vi "Read Thermocouples and Voltages v181004_A.vi"() -> ()   [LabVIEW 2017]
doc: "I. Description:\nThis example demonstrates how to make continuous, hardware-timed temperature measurement using a thermocouple.\n\nII. Instructions for Running:\n1. Specify the Physical Channel where you have connected the thermocouple.\n2. Enter the Minimum and Maximum temperature values in degrees C you expect to measure. A smaller range will allow a more accurate measurement.\n3. Enter the scan rate at which you want to run the acquisition.\n4. Specify the type of thermocouple you are using.\n5. Thermocouple measurements require cold-junction compensation (CJC) to correctly scale them. Specify the source of your cold-junction compensation.\n6. If your CJC source is \"Internal\", skip the rest of the steps.\n7. If your CJC source is \"Constant Value\", specify the value (usually room temperature) in degrees C.\n8. If your CJC source is \"Channel\", specify the CJC Channel name. \n9. Specify the appropriate Auto Zero Mode. See your device's hardware manual to find out if your device supports this attribute.\n\nIII. Block Diagram Steps:\n1. Create a Thermocouple (TC) temperature measurement channel.\n2. Get all the channels in the task.\n3. Convert channel(s) array to a comma-delimited channel string.\n4. This attribute is set to compensate for input offset errors. May not be supported by all devices*.\n5. Call the Timing VI to specify the hardware timing parameters. Use device's internal clock, continuous mode acquisition and the sample rate specified by the user.\n6. Call the Start VI to program and start the acquisition.\n7. Read N samples and plot it. By default, the Read VI reads all available samples, but you can specify how many samples to read at a time and the timeout value. Continue reading data until the stop button is pressed or an error occurs. \n8. Call the Clear Task VI to clear the Task.\n9. Use the popup dialog box to display an error if any.\n\n* If your device does not support Auto Zero Mode bypass Step 2, 3, and 4.\n\nIV. I/O Connections Overview:\nConnect your thermocouple to the terminals corresponding to the Physical Channel I/O Control value."
uses:
  <vilib>/Utility/error.llb/DialogType.ctl
  <vilib>/DAQmx/read.llb/DAQmx Read (Counter 1D DBL 1Chan NSamp).vi
  <vilib>/Analysis/baseanly.llb/Mean (DBL).vi
  <vilib>/DAQmx/write.llb/DAQmx Write (Digital 1D Bool NChan 1Samp 1Line).vi
  <vilib>/DAQmx/read.llb/DAQmx Read (Analog 1D Wfm NChan NSamp).vi
  <vilib>/DAQmx/create/channels.llb/DAQmx Create Channel (AI-Voltage-Basic).vi
  <vilib>/DAQmx/configure/timing.llb/DAQmx Timing (Sample Clock).vi
  <vilib>/DAQmx/create/channels.llb/DAQmx Create Channel (DO-Digital Output).vi
  <vilib>/Waveform/WDTOps.llb/WDT Index Channel DBL.vi
  <vilib>/DAQmx/miscellaneous.llb/DAQmx Fill In Error Info.vi
  <vilib>/DAQmx/create/channels.llb/DAQmx Create Channel (CI-Period).vi
  <vilib>/DAQmx/configure/timing.llb/DAQmx Timing (Implicit).vi
  <vilib>/express/express arith-compare/Formula/XNode/ExpressFormulaBlockNode.xnode
  <resource>/objmgr/daqmx.rc
  <vilib>/Analysis/NI_AALBase.lvlib
  <vilib>/ptbypt/NI_PtbyPt.lvlib
panel:
  out "TRQ_T22_2SPD_INPUT_PULLEY":dbl=0.017996215820312494 format="%0.3f"
  in  "offset_TRQ_IN":dbl=-0.15 format="%5.2f"
  in  "(N·m)/V TRQ_IN":dbl=20.0 format="%5.2f"
  in  "CI.Period.DigFltr.MinPulseWidth":dbl=1e-05 format="%.3e"
  out "CALC_RPM_2SPD_IN_FV":dbl=3496.0559999999996 format="%0.1f"
  out "T2":dbl=102.18860626220703 format="%0.3f"
  in  "offset_T2":dbl=-50.0 format="%5.3f"
  in  "T2 °C/V":dbl=50.0 format="%5.3f"
  in  "offset RPM_IN":dbl=4.0 format="%5.2f"
  in  "RPM_OT/V":dbl=2803.738 format="%5.3f"
  out "RPM_2SPD_IN_FV":dbl=1.4714915466308593 format="%0.1f"
  in  "offset TRQ_OT":dbl format="%5.2f"
  in  "N·m/V":dbl=10.0 format="%5.2f"
  out "TRQ_2SPD_OT (N·m)":dbl=-0.0037994384765625 format="%0.3f"
  out "Power_OT (W)":dbl=-0.0009464121851047188 format="%.2f"
  in  "Physical Channel 2":tag="Dev2/ai0:7" caption="PCI-6143_2 Channels"
  out "rpm_out/rpm_in":dbl=1.6164955643487515 format="%.3g"
  out "switch_counts":dbl=4500000.0
  in  "switch_time (s)":dbl=900000.0
  out "AI Consumer Iterations":i32=21
  out "Counter Consumer":i32=248
  out "Counter Producer":i32=247
  out "PPR":i32=107
  out "Array":dbl[](array[numeric])
  out "Mean RPM_2SPD_OT":dbl
  out "data":dbl[][](array[numeric])
  in  "LV_CMD_2SPD_OIL_SLND":bool[](array[boolean])=[FALSE]
  in  "lines":tag="Dev1/port0/line0"
  out "RPM_2SPD_OT_6602":dbl format="%0.1f"
  in  "PPR Array":i32[](array[numeric])=[360, 107]
  in  "CI.Counter":tag[](array[tag])=["Dev3/ctr0", "Dev3/ctr1"]
  in  "CI.Period.Terminal":tag[](array[tag])=["/Dev3/PFI1", "/Dev3/PFI38"]
  in  "path":path=path "\\\\Achates.lan\\data/TeamShares/Testing Group/Bench Tests/PR22093 - Orthrus 2SpdSN3.4 Sprag Clutch durability testing/LabView Data"
  in  "DRVLN_PULLEY_RATIO":dbl=1.48 format="%.2f"
  out "delta-P":dbl=2.3032233810424803 format="%.3f"
  in  "F2 gpm/V":dbl=0.875 format="%5.3f"
  out "F2":dbl=0.5424336433410645 format="%0.3f"
  in  "offset_F2":dbl=-0.875 format="%5.3f"
  out "Recorded Blocks":dbl=-95911.0
  out "AI Producer Iterations":i32=20
  in  "Force Record":bool caption="Force Record Enable"
  out "RPM_DRVLN_6602":dbl format="%0.1f"
  in  "offset_RPM1":dbl format="%5.3f"
  in  "RPM_IN rpm/V":dbl=2362.2 format="%5.3f"
  out "RPM_2SPD_OT_FV":dbl=2.3786595581054684 format="%0.1f"
  in  "offset_T1":dbl=-50.0 format="%5.3f"
  in  "T1 °C/V":dbl=50.0 format="%5.3f"
  out "T1":dbl=104.08489227294922 format="%0.3f"
  out "P3":dbl=3.2324594879150386 format="%0.3f"
  in  "offset_P3":dbl=0.01 format="%5.3f"
  in  "P3 bar_g/V":dbl=2.05 format="%5.3f"
  out "P2":dbl=3.3167593002319333 format="%0.3f"
  in  "offset_P2":dbl format="%5.3f"
  in  "P2 bar_a/V":dbl=2.05 format="%5.3f"
  out "P1":dbl=1.013535919189453 format="%0.3f"
  in  "offset_P1":dbl=-0.01 format="%5.3f"
  in  "P1 bar_a/V":dbl=1.0 format="%5.3f"
  out "data 2":waveform(dbl)[](array[waveform])=[{"t0"=timestamp(3621514488.0231304 s since 1904-01-01), "dt"=0.1, "Y"=[-0.0004058837890625, 0.0021026611328125], "attributes"=variant("NI_ChannelName"=variant(string "Dev1/ai0"), "NI_UnitDescription"=variant(string "Volts"))}, {"t0"=timestamp(3621514488.0231304 s since 1904-01-01), "dt"=0.1, "Y"=[1.0246047973632812, 1.022467041015625], "attributes"=variant("NI_ChannelName"=variant(string "Dev1/ai0"), "NI_UnitDescription"=variant(string "Volts"))}, {"t0"=timestamp(3621514488.0231304 s since 1904-01-01), "dt"=0.1, "Y"=[1.6239944458007813, 1.6118682861328124], "attributes"=variant("NI_ChannelName"=variant(string "Dev1/ai0"), "NI_UnitDescription"=variant(string "Volts"))}, {"t0"=timestamp(3621514488.0231304 s since 1904-01-01), "dt"=0.1, "Y"=[1.5774093627929688, 1.5664535522460938], "attributes"=variant("NI_ChannelName"=variant(string "Dev1/ai0"), "NI_UnitDescription"=variant(string "Volts"))}, {"t0"=timestamp(3621514488.0231304 s since 1904-01-01), "dt"=0.1, "Y"=[3.0814483642578123, 3.0819473266601562], "attributes"=variant("NI_ChannelName"=variant(string "Dev1/ai0"), "NI_UnitDescription"=variant(string "Volts"))}, {"t0"=timestamp(3621514488.0231304 s since 1904-01-01), "dt"=0.1, "Y"=[1.62095947265625, 1.6188888549804688], "attributes"=variant("NI_ChannelName"=variant(string "Dev1/ai0"), "NI_UnitDescription"=variant(string "Volts"))}, {"t0"=timestamp(3621514488.0231304 s since 1904-01-01), "dt"=0.1, "Y"=[-0.018182373046875, -0.01845550537109375], "attributes"=variant("NI_ChannelName"=variant(string "Dev1/ai0"), "NI_UnitDescription"=variant(string "Volts"))}, {"t0"=timestamp(3621514488.0231304 s since 1904-01-01), "dt"=0.1, "Y"=[-0.00205078125, -9.002685546875e-05], "attributes"=variant("NI_ChannelName"=variant(string "Dev1/ai0"), "NI_UnitDescription"=variant(string "Volts"))}, {"t0"=timestamp(3621514488.0231304 s since 1904-01-01), "dt"=0.1, "Y"=[0.00018768310546875, -0.00094757080078125], "attributes"=variant("NI_ChannelName"=variant(string "Dev1/ai0"), "NI_UnitDescription"=variant(string "Volts"))}, {"t0"=timestamp(3621514488.0231304 s since 1904-01-01), "dt"=0.1, "Y"=[3.0438766479492188, 3.0436676025390623], "attributes"=variant("NI_ChannelName"=variant(string "Dev1/ai0"), "NI_UnitDescription"=variant(string "Volts"))}, {"t0"=timestamp(3621514488.0231304 s since 1904-01-01), "dt"=0.1, "Y"=[-0.001458740234375, 0.0050140380859375], "attributes"=variant("NI_ChannelName"=variant(string "Dev1/ai0"), "NI_UnitDescription"=variant(string "Volts"))}, {"t0"=timestamp(3621514488.0231304 s since 1904-01-01), "dt"=0.1, "Y"=[-0.00649566650390625, -0.0067047119140625], "attributes"=variant("NI_ChannelName"=variant(string "Dev1/ai0"), "NI_UnitDescription"=variant(string "Volts"))}, {"t0"=timestamp(3621514488.0231304 s since 1904-01-01), "dt"=0.1, "Y"=[-0.10598602294921874, -0.10598602294921874], "attributes"=variant("NI_ChannelName"=variant(string "Dev1/ai0"), "NI_UnitDescription"=variant(string "Volts"))}, {"t0"=timestamp(3621514488.0231304 s since 1904-01-01), "dt"=0.1, "Y"=[-1.2560470581054688, -1.25604248046875], "attributes"=variant("NI_ChannelName"=variant(string "Dev1/ai0"), "NI_UnitDescription"=variant(string "Volts"))}, {"t0"=timestamp(3621514488.0231304 s since 1904-01-01), "dt"=0.1, "Y"=[-0.90093994140625, -0.90093994140625], "attributes"=variant("NI_ChannelName"=variant(string "Dev1/ai0"), "NI_UnitDescription"=variant(string "Volts"))}, {"t0"=timestamp(3621514488.0231304 s since 1904-01-01), "dt"=0.1, "Y"=[-0.12911529541015626, -0.129156494140625], "attributes"=variant("NI_ChannelName"=variant(string "Dev1/ai0"), "NI_UnitDescription"=variant(string "Volts"))}]
  out "Power_IN (W)":dbl=0.002773113099357126 format="%.2g"
  out "error out":errorcluster
  in  "error in (no error)":errorcluster
  out "Mean RPM_DRVLN":dbl
  out "TRQ_2SPD_DRVLN_OT (N·m)":dbl=-0.026378784179687476 format="%0.3f"
  in  "(N·m)/V DRVLN":dbl=20.0 format="%5.2f"
  in  "offset_TRQ_DRVLN":dbl=0.34 format="%5.2f"
  out "Waveform Chart":waveform(dbl)[](graph)=[{"t0"=timestamp(3621514488.0231304 s since 1904-01-01), "dt"=0.1, "Y"=[0.0018768310546875, -0.0094757080078125], "attributes"=variant("NI_ChannelName"=variant(string "TRQ_2SPD_OT"), "NI_UnitDescription"=variant(string "N·m"))}, {"t0"=timestamp(3621514488.0231304 s since 1904-01-01), "dt"=0.1, "Y"=[-0.8443554687499999, 3.7873385620117186], "attributes"=variant("NI_ChannelName"=variant(string "RPM_2SPD_IN_FV"), "NI_UnitDescription"=variant(string "rpm"))}, {"t0"=timestamp(3621514488.0231304 s since 1904-01-01), "dt"=0.1, "Y"=[-0.023647460937499976, -0.029110107421874976], "attributes"=variant("NI_ChannelName"=variant(string "TRQ_2SPD_DRVLN_OT"), "NI_UnitDescription"=variant(string "N·m"))}, {"t0"=timestamp(3621514488.0231304 s since 1904-01-01), "dt"=0.1, "Y"=[1.0146047973632812, 1.012467041015625], "attributes"=variant("NI_ChannelName"=variant(string "P_2SPD_VENT"), "NI_UnitDescription"=variant(string "bar_a"))}, {"t0"=timestamp(3621514488.0231304 s since 1904-01-01), "dt"=0.1, "Y"=[3.3291886138916014, 3.3043299865722653], "attributes"=variant("NI_ChannelName"=variant(string "P_OIL_2SPD_IN"), "NI_UnitDescription"=variant(string "bar_a"))}, {"t0"=timestamp(3621514488.0231304 s since 1904-01-01), "dt"=0.1, "Y"=[3.2436891937255856, 3.221229782104492], "attributes"=variant("NI_ChannelName"=variant(string "P_OIL_2SPD_SLND_OT"), "NI_UnitDescription"=variant(string "bar_a"))}, {"t0"=timestamp(3621514488.0231304 s since 1904-01-01), "dt"=0.1, "Y"=[104.07241821289062, 104.09736633300781], "attributes"=variant("NI_ChannelName"=variant(string "T_2SPD_OIL_IN"), "NI_UnitDescription"=variant(string "deg_C"))}, {"t0"=timestamp(3621514488.0231304 s since 1904-01-01), "dt"=0.1, "Y"=[102.19383239746094, 102.18338012695312], "attributes"=variant("NI_ChannelName"=variant(string "T_2SPD_OIL_OT"), "NI_UnitDescription"=variant(string "deg_C"))}, {"t0"=timestamp(3621514488.0231304 s since 1904-01-01), "dt"=0.1, "Y"=[0.020086669921874994, 0.015905761718749994], "attributes"=variant("NI_ChannelName"=variant(string "TRQ_T22_2SPD_INPUT_PULLEY"), "NI_UnitDescription"=variant(string "N·m"))}, {"t0"=timestamp(3621514488.0231304 s since 1904-01-01), "dt"=0.1, "Y"=[-1.1379918029785157, 5.895310919189453], "attributes"=variant("NI_ChannelName"=variant(string "RPM_2SPD_OT_FV"), "NI_UnitDescription"=variant(string "rpm"))}, {"t0"=timestamp(3621514488.0231304 s since 1904-01-01), "dt"=0.1, "Y"=[0.0, 0.0], "attributes"=variant("NI_ChannelName"=variant(string "RPM_DRVLN_6602"), "NI_UnitDescription"=variant(string "rpm"))}, {"t0"=timestamp(3621514488.0231304 s since 1904-01-01), "dt"=0.1, "Y"=[0.0, 0.0], "attributes"=variant("NI_ChannelName"=variant(string "RPM_2SPD_OT_6602"), "NI_UnitDescription"=variant(string "rpm"))}, {"t0"=timestamp(3621514488.0231304 s since 1904-01-01), "dt"=0.1, "Y"=[0.5433395385742188, 0.5415277481079102], "attributes"=variant("NI_ChannelName"=variant(string "VFr_OIL_2SPD_IN"), "NI_UnitDescription"=variant(string "gpm"))}, {"t0"=timestamp(3621514488.0231304 s since 1904-01-01), "dt"=0.1, "Y"=[1.6164955643487515, 1.6164955643487515], "attributes"=variant("NI_ChannelName"=variant(string "RPM_RATIO"), "NI_UnitDescription"=variant(string "ratio"))}, {"t0"=timestamp(3621514488.0231304 s since 1904-01-01), "dt"=0.1, "Y"=[99.0, 99.0], "attributes"=variant("NI_ChannelName"=variant(string "DataTag"), "NI_UnitDescription"=variant(string "none"))}, {"t0"=timestamp(3621514488.0231304 s since 1904-01-01), "dt"=0.1, "Y"=[0.0, 0.0], "attributes"=variant("NI_ChannelName"=variant(string "LV_CMD_2SPD_OIL_SLND"), "NI_UnitDescription"=variant(string "boolean"))}]
  in  "Run Letter":string="a"
  out "Recording":bool
  in  "Num_Blocks":dbl=100.0
  in  "Data Tag":dbl=99.0 format="%.2p"
  in  "Maximum Value":dbl=5.0 format="%0.2f"
  in  "Minimum Value":dbl=-5.0 format="%0.2f"
  in  "Physical Channel":tag="Dev1/ai0:7" caption="PCI-6143_1 Channels"
  in  "stop":bool
  in  "Rate":dbl=1000.0 format="%0.2f"
  # "rev 150415_A  added \"Record Run X\" sub VI.\nrev 150423_A added power, efficiency, and manual inputs for speed .\nrev 150423_B added speed measurement via PCI-6602 card.\nrev 161117_A is set up for the alternator test reading shaft RPM from Dynapar encoder and torque from the Omega TQ513-1K paired with the Omega DP41-S.\nrev 170504_A migrated DAQ h/w from the SCXI chassis (now being used for TC2 porcupine testing) to PCI-6143.\nrev 170510_A takes data at 1000Hz, then averages groups of 100 samples for a logging rate of 10Hz per channel.  Added function that resets \"Data Tag\"\nto 99 after \"Num_Blocks\" has been recorded.\nrev 170810_A adds flowmeter for 2-speed supercharger drive bench test.  CJP\nrev 170821_A logs tags to same file for a given run letter.  Uses \"Record Continuous Tags...\" sub VI.\nrev 171129_A is for the Orthrus 2-speed drive.  Added new encoder period measurement for the 127 tooth geat \"RPM_2SPD_OT\". CJP\nrev 171130_A adds Digital Output (DO) for 2SPD drive control.  Will log this with the rest of the data.  Also corrected the number of teeth on the 2SPD Output side from 127 to 107!\nrev 171201_A restructuring for  \"real-time\" response to speed changes by moving the disklog to a separate loop (queue).\nrev 171201_B moves counters into main AI loop and adds a start trigger so DAQ won't start until rig is spinning.  Added F-V where old \"F1\" channel was for \"RPM_2SPD_OT\".   CJP\nrev 171201_C uses a CI-Frequency task for RPM instead of period.  Testing this for better transient response.  This appears to be even slower than the period measurement.\nrev 171201_D is built from rev 171201_A, but adding in the F-V channel.  This version queues both the AI channel and CI channels to a single Consumer.  Also adding a 30s switch to automate switching of the 2SPD solenoid.\nrev 171221_A was the first attempt at this and for some reason, while running that VI, the computer froze, unable to do ctrl+alt+del reboot.  After rebooting, the VI was no longer openable in LabView 2014 or LabView 2016.  Will try the same process over with v171226_A.\nrev 171226_A adds one more PCI_6143 card for 8 additional analog inputs.\nrev 171226_B created a backup with 171226_A.\nrev 180314_A added thermocouple for Sumanth.  This is for testing the 2-Speed Drive.\nrev Read \"ThermVolt_TestSpeed_180406_A.vi\" is for verifying the one remaining Micro-Epsilon speed sensor on the 2Spd Drive.\nrev \"Read Thermocouples and Voltages v180406_A.vi\" reintroduces the two counter/timer channels on the PCI-6602 card for the driveline encoder and \nMicro-Epsilon 2Spd Output.\nrev 180919_A built off of rev 180426_A for 2-Speed Drive testing.  CJP\nv181002_A adding new T22 at 2SPD input pulley AND keeping original T22 at output end of drivline.  CJP\nv181004_A corrected front panel displays for Power_IN and Power_OT.  CJP"
  # "HBM T21WN"
  # "Interface T22"
  # "For instructions, select Help>>Show Context Help"
  # "Timing Parameters"
  # "Now using 360 PPR encoder for input speed 171227.\nChanged to Input Gear Speed 180118.  CJP  127 Hz = 1 RPS, 127 Hz = 60 RPM\n5 kHz = 1 V => 5000/127 = 39.37 RPS = 2362.205 RPM\nv180314_A 5kHz = 1V = 5000/360 = 13.888 RPS = 833.33 RPM.\nBack to 360PPR encoder with pulley ratio of 1.48."
  # "P1 is 0-5 bar a sensor with 0-10V output giong to voltage divider,\nso PCI-6143 reads 0-2.5 bar a."
  # "Changed to \"P_2SPD_Vent\" 171229.   P_OIL_2SPD_LAYSHAFT\n0-5 bar a sensor through 5B module (±10V input to ±5V output)"
  # "P_OIL_2SPD_IN"
  # "P_OIL_2SPD_SLND_OT"
  # "T_2SPD_OIL_IN"
  # "T_2SPD_OIL_OT"
  # "Hoffer SN168754, 0-3.5 gpm = 4-20 mA = 1-5 VDC (v171226_B)"
  # "Was 1.23 in v171201_D, changed to 1.48 in v171226_A."
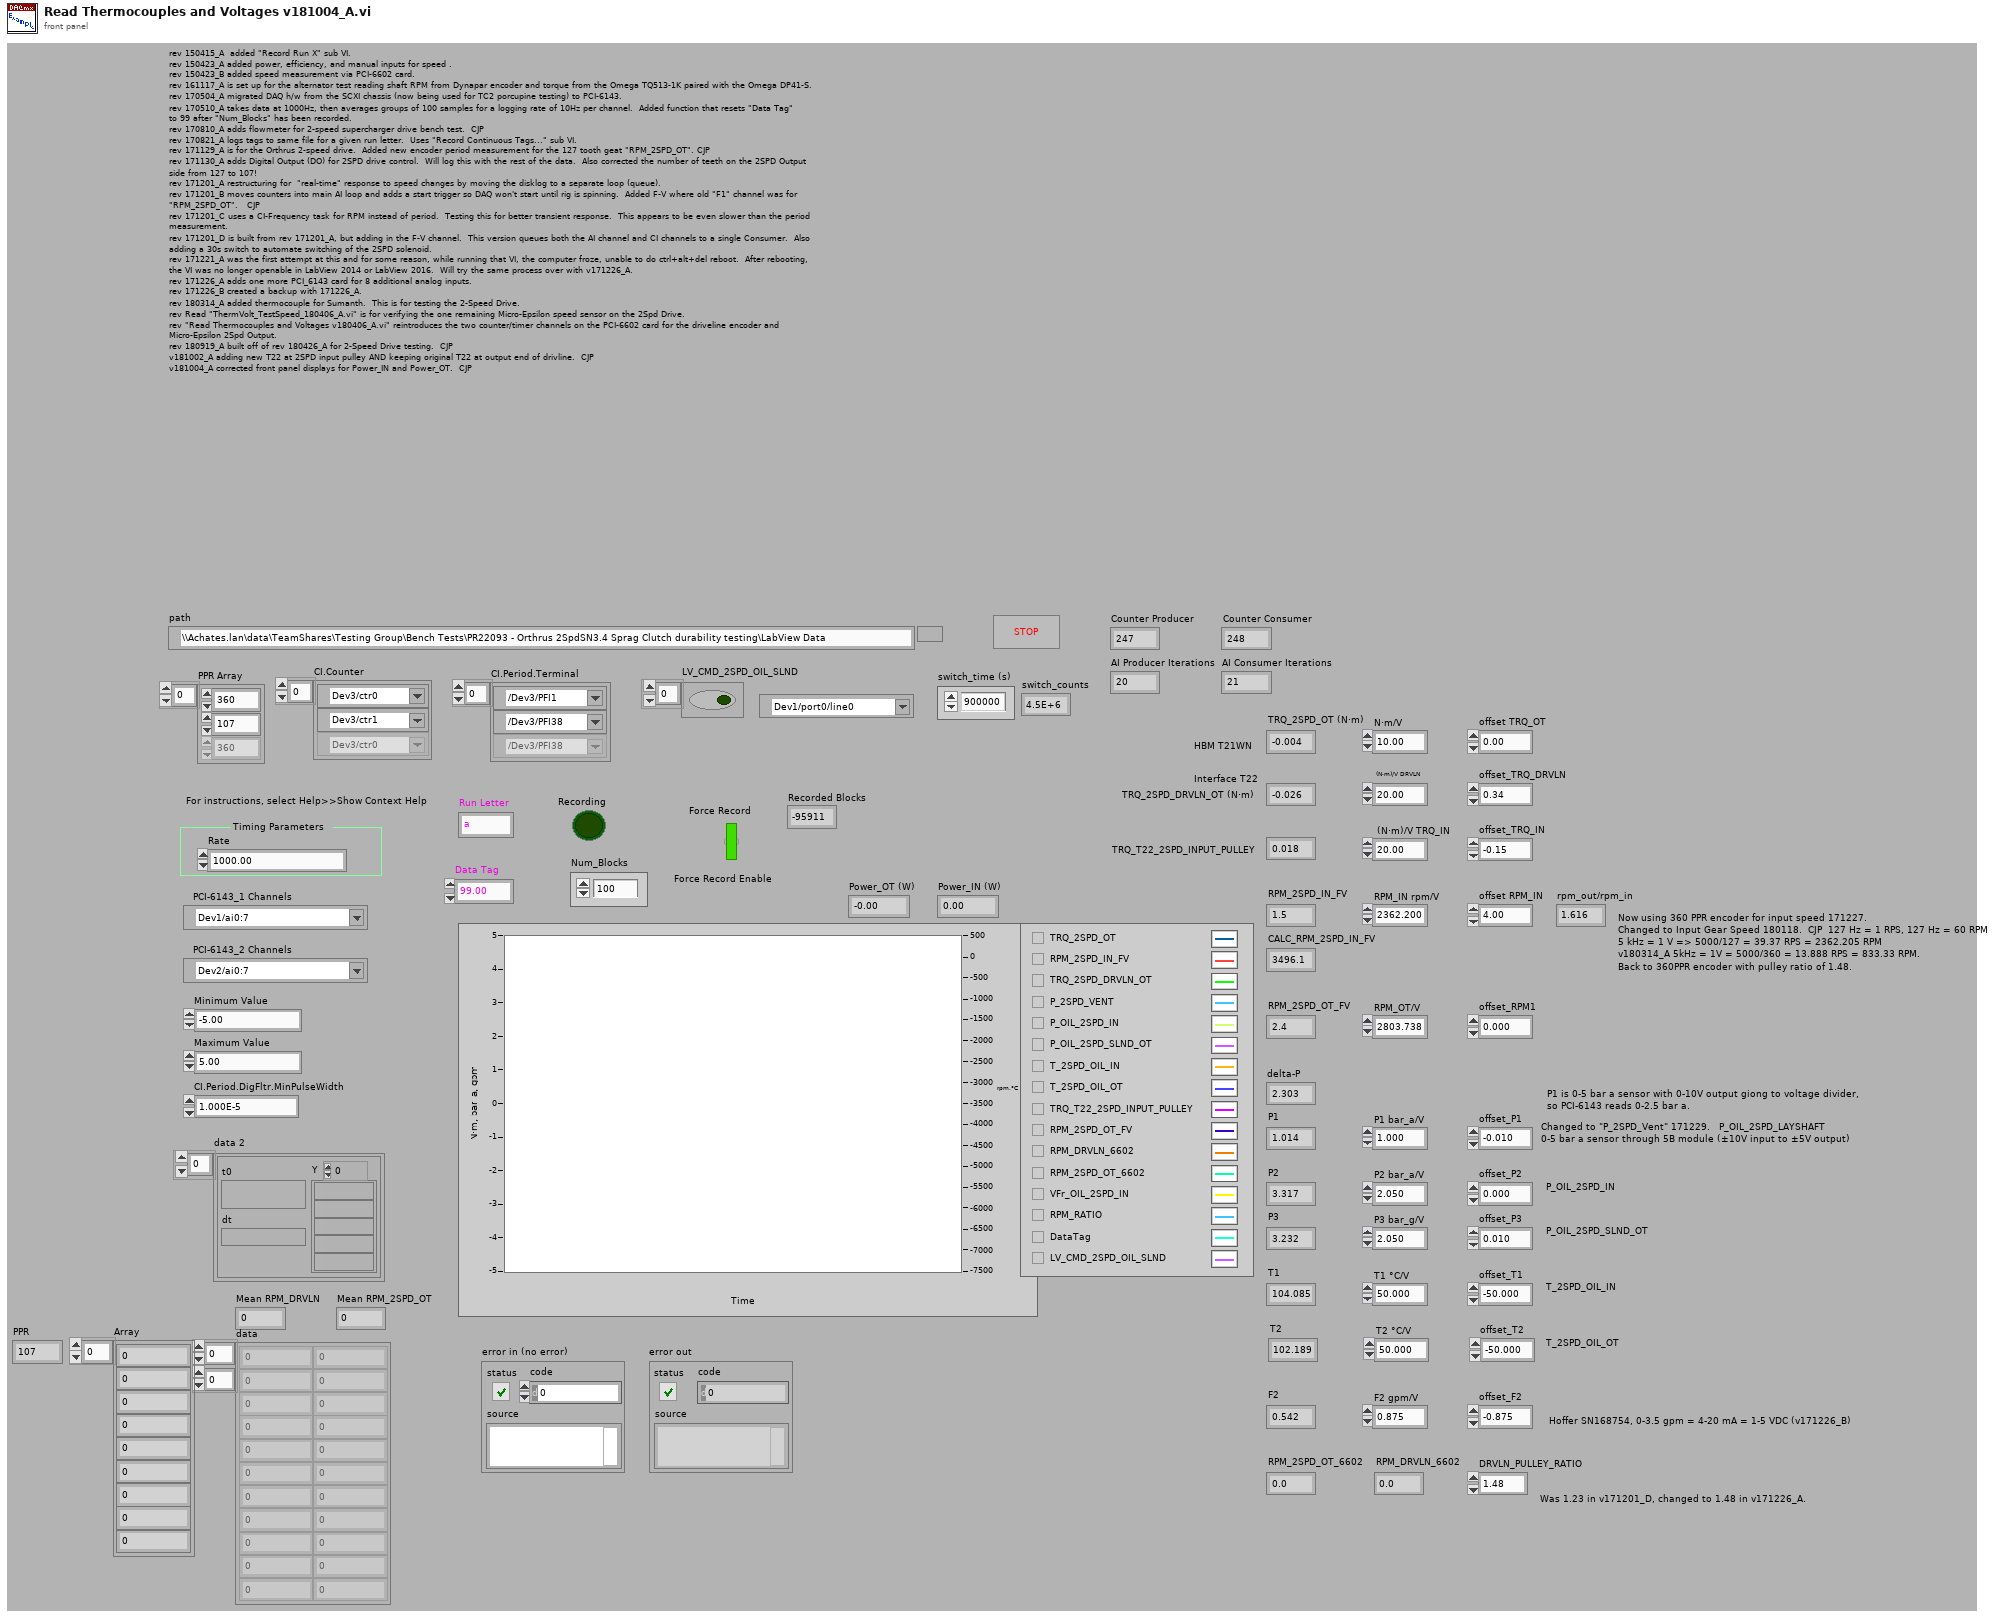
[diagram p1: front panel]
types:
  T1 = typedef "DialogType.ctl" = u16
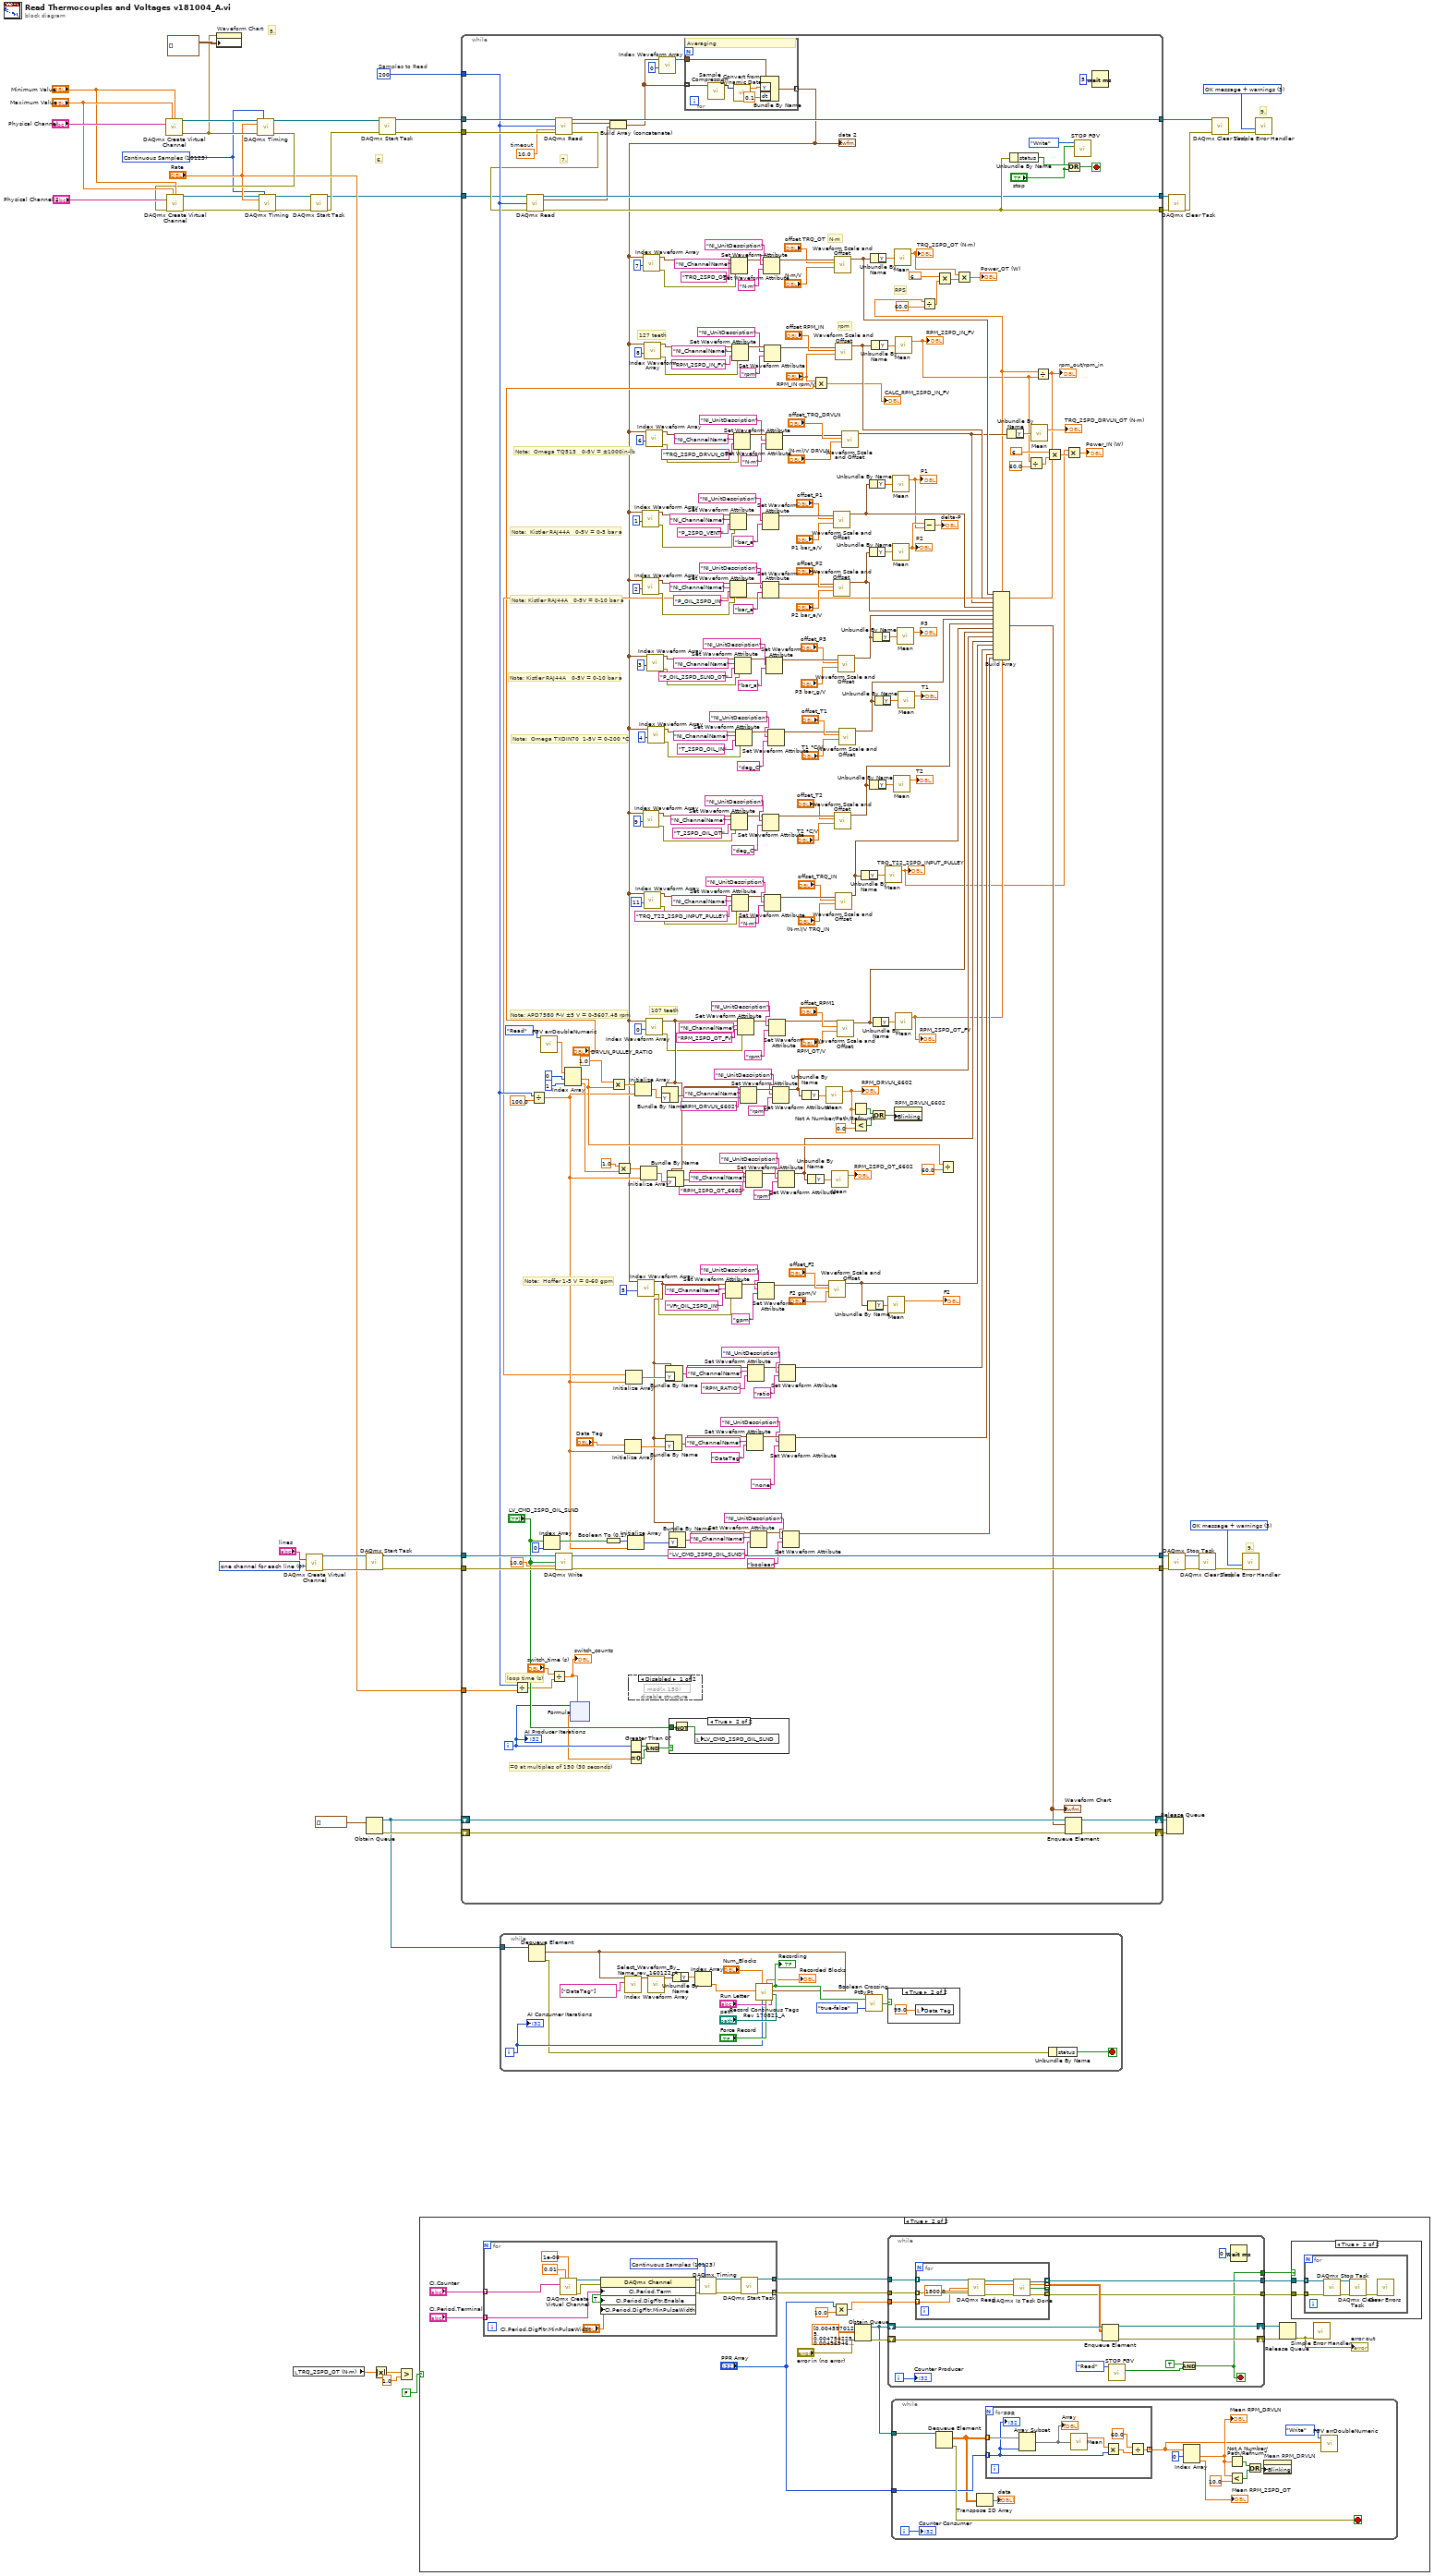
[diagram p0: block diagram]
diagram:
  w27 = T1 3 items=["no dialog", "OK message", "continue or stop message", "OK message + warnings", "continue/stop + warnings"] ("type of dialog (OK msg:1)")
  w33 = 0 items=["one channel for each line", "one channel for all lines"] ("line grouping")
  w42 = T1 3 items=["no dialog", "OK message", "continue or stop message", "OK message + warnings", "continue/stop + warnings"] ("type of dialog (OK msg:1)")
  w11 = 10123 items=["Finite Samples"=10178, "Continuous Samples"=10123] ("sample mode")
  # "Samples to Read"
  # "9."
  # "9."
  # "5."
  # "6."
  n1 = call-poly <vilib>:"DAQmx Create Virtual Channel.vi"("maximum value"="Maximum Value", "minimum value"="Minimum Value", "physical channels"="Physical Channel") -> ("task out"=w40:refnum<k21>, "error out"=w37:errorcluster)  [unwired: 11 in]
  n2 = property on="Waveform Chart" class="WFChart (strict)"(error in=w37, "History Data"=waveform(dbl)[][] []) -> ()  [unwired: 1 in, 2 out]
  n3 = call-poly <vilib>:"DAQmx Timing.vi"("task/channels in"=w40, "sample mode"=w11, "rate"="Rate", "error in"=w37) -> ("task out"=w43:refnum<k21>, "error out"=w13:errorcluster)  [unwired: 10 in]
  n4 = call-poly <vilib>:"DAQmx Create Virtual Channel.vi"("maximum value"="Maximum Value", "minimum value"="Minimum Value", "physical channels"="Physical Channel 2", "error in"=w13) -> ("task out"=w10:refnum<k21>, "error out"=w9:errorcluster)  [unwired: 10 in]
  n5 = call-poly <vilib>:"DAQmx Timing.vi"("task/channels in"=w10, "sample mode"=w11, "rate"="Rate", "error in"=w9) -> ("task out"=w8:refnum<k21>, "error out"=w7:errorcluster)  [unwired: 10 in]
  n6 = local read "TRQ_2SPD_OT (N·m)"() -> (w36:dbl)
  n7 = call-poly <vilib>:"DAQmx Create Virtual Channel.vi"("lines"="lines", "line grouping"=w33) -> ("task out"=w32:refnum<k21>, "error out"=w31:errorcluster)  [unwired: 12 in]
  n8 = call <vilib>:"DAQmx Start Task.vi"("task/channels in"=w8, "error in"=w7) -> ("task out"=w2:refnum<k21>, "error out"=w6:errorcluster)  [unwired: 12 in]
  n9 = call <vilib>:"DAQmx Start Task.vi"("task/channels in"=w32, "error in"=w31) -> ("task out"=w30:refnum<k21>, "error out"=w29:errorcluster)  [unwired: 12 in]
  n10 = Obtain Queue(element data type=waveform(dbl)[] [] ("appended array")) -> (queue out=w17:refnum<queue>, error out=w20:errorcluster)  [unwired: 4 in, 1 out]
  n11 = Absolute Value(x=w36) -> (abs(x)=w35:dbl)
  n12 = call <vilib>:"DAQmx Start Task.vi"("task/channels in"=w43, "error in"=w6) -> ("task out"=w45:refnum<k21>, "error out"=w46:errorcluster)  [unwired: 12 in]
  n13 = Greater?(x=w35, y=1.0) -> ()  [unwired: 1 out]
  n14 = case shown="True" FALSE ("x > y?") {
    frame False {
    }
    frame True {
      n15 = for {
        tunnel: "CI.Counter" -> [w79] mode=indexing
        tunnel: "CI.Period.Terminal" -> [w78] mode=indexing
        tunnel: [w75] -> w53 mode=indexing
        tunnel: [w74] -> w52 mode=indexing
        w82 = 10123 items=["Finite Samples"=10178, "Continuous Samples"=10123, "Hardware Timed Single Point"=12522] ("sample mode")
        n16 = call-poly <vilib>:"DAQmx Create Virtual Channel.vi"("maximum value"=0.01, "minimum value"=1e-06, "counter"=w79) -> ("task out"=w86:refnum<k21>, "error out"=w85:errorcluster)  [unwired: 11 in]
        n17 = property class="DAQmx Channel"(reference=w86, error in=w85, "CI.Period.Term"=w78, "CI.Period.DigFltr.Enable"=TRUE, "CI.Period.DigFltr.MinPulseWidth"="CI.Period.DigFltr.MinPulseWidth") -> (reference out=w81:refnum<k21>, error out=w80:errorcluster)
        n18 = call-poly <vilib>:"DAQmx Timing.vi"("task/channels in"=w81, "sample mode"=w82, "error in"=w80) -> ("task out"=w77:refnum<k21>, "error out"=w76:errorcluster)  [unwired: 11 in]
        n19 = call <vilib>:"DAQmx Start Task.vi"("task/channels in"=w77, "error in"=w76) -> ("task out"=w75:refnum<k21>, "error out"=w74:errorcluster)  [unwired: 12 in]
      }
      n20 = Multiply(x="PPR Array", y=10.0) -> (x*y=w48:dbl[])
      n21 = Obtain Queue(element data type=dbl[][] [[0.0045970125, 0.004754225, 0.0049694625, 0.0050692375, 0.0053127875, 0.0054311125, 0.0055065625, 0.0056537374999999996, 0.005769887499999999, 0.005887074999999999, 0.006048225, 0.006217149999999999, 0.00639135, 0.006574549999999999, 0.00679575, 0.0070303625, 0.007265524999999999, 0.007534175, 0.00788215, 0.0083976625, 0.0090313125, 0.0099294625, 0.0107609875, 0.011527774999999999, 0.012710349999999999, 0.0140843875, 0.016087512499999998, 0.0192914, 0.026565025, 0.049202687499999995, 0.0411767125, 0.027019124999999998, 0.0193940875, 0.014989537499999999, 0.0125112625, 0.0108602875, 0.009911375, 0.0090453125, 0.008389275, 0.0079261625, 0.007504537499999999, 0.007138475, 0.0068520874999999995, 0.00661185, 0.0063869625, 0.006171962499999999, 0.0059779375, 0.0058176, 0.005667274999999999, 0.005517874999999999, 0.0053826874999999995, 0.0052555499999999995, 0.005129587499999999, 0.0050265375, 0.0049228875, 0.0048274749999999995, 0.0047371125, 0.0046559374999999995, 0.0045791375, 0.004499537499999999, 0.0044337375, 0.004377625, 0.0043221625, 0.0042752125, 0.00423415, 0.0041989374999999995, 0.004174225, 0.0041491374999999995, 0.0041306625, 0.0041195, 0.0041102874999999995, 0.0041087125, 0.0041085, 0.0041173625, 0.0041233875, 0.00414, 0.0041636, 0.004193425, 0.0042221125, 0.0042557125, 0.0043001624999999995, 0.0043338874999999995, 0.004381075, 0.0044340125, 0.0044918499999999995, 0.0045553625, 0.00461945, 0.004695425, 0.0047688125, 0.004849475, 0.0049211624999999995, 0.0050037875, 0.0050873624999999995, 0.00517665, 0.0052699625, 0.0053783749999999995, 0.0055095, 0.0056566375, 0.0059320375, 0.0061901125, 0.0064714874999999995, 0.006735425, 0.0069463625, 0.0071708499999999994, 0.0074100875, 0.007671462499999999, 0.007957724999999999, 0.008274749999999999, 0.008649612499999999, 0.009184099999999999, 0.0100510125, 0.011108999999999999, 0.012166825, 0.013310975, 0.0149006625, 0.0171997375, 0.0214567375, 0.045855799999999995, 0.09502265, 0.020254875, 0.0141139875, 0.0111827, 0.009689775, 0.0082998, 0.0074224124999999995, 0.006898262499999999, 0.006426512499999999, 0.005930749999999999, 0.00551425, 0.0052099124999999994, 0.005005875, 0.004816625, 0.0046209125, 0.004423825, 0.0042374249999999995, 0.004093625, 0.003980249999999999, 0.0038957749999999998, 0.003813675, 0.0037337125, 0.0036417625, 0.0035518, 0.0034750249999999996, 0.0034133625, 0.0033704, 0.0033326999999999996, 0.0033086624999999997, 0.0032780875, 0.0032493125, 0.0032172625, 0.0031830125, 0.003156075, 0.0031351, 0.0031223124999999997, 0.0031195625, 0.0031195999999999997, 0.0031262875, 0.0031262625, 0.0031187625, 0.003112175, 0.0031013, 0.0031000625, 0.0031061749999999996, 0.0031148375, 0.0031363124999999998, 0.0031575875, 0.0031793374999999997, 0.0031989375, 0.003209375, 0.0032187749999999997, 0.0032246749999999998, 0.0032393499999999998, 0.0032596375, 0.0032846999999999998, 0.0033129875, 0.0033398875, 0.0033605625, 0.0033730125, 0.0033800625, 0.0033910374999999997, 0.0034024999999999997, 0.0034324499999999997, 0.0034692125, 0.003487375, 0.0036092, 0.0036641374999999998, 0.00375065, 0.00382645, 0.003900275, 0.0039815499999999995, 0.00401405, 0.0041001, 0.004137, 0.004206275, 0.0042273625, 0.004273175, 0.004318499999999999, 0.0043875875, 0.004465937499999999, 0.00454645, 0.0046162875, 0.0046560125, 0.004719375, 0.004783524999999999, 0.00488935, 0.0050024375, 0.005090737499999999, 0.005181725, 0.005256662499999999, 0.0054578249999999995, 0.005663525, 0.0059690375, 0.0062521, 0.0064150249999999995, 0.0066076, 0.0069134875, 0.0072418874999999995, 0.007530512499999999, 0.00789695, 0.0084488125, 0.009043325, 0.0096281375, 0.010537325, 0.0117254875, 0.0131475625, 0.016035024999999998, 0.021346762499999998, 0.035288475, 0.02836915, 0.0214058375, 0.0158160125, 0.012597962499999999, 0.010421375, 0.0091907125, 0.008092199999999999, 0.007308149999999999, 0.006767975, 0.00628305, 0.00585645, 0.005523525, 0.00526055, 0.0050496125, 0.0048642749999999995, 0.0046817125, 0.004526925, 0.0043958, 0.0042943625, 0.0042028625, 0.0041157625, 0.0040372624999999995, 0.0039606625, 0.0038940374999999997, 0.0038366625, 0.00378715, 0.0037529125, 0.0037186, 0.0036958499999999997, 0.003675125, 0.003658575, 0.0036452625, 0.0036209124999999997, 0.003620525, 0.0036184625, 0.0036254875, 0.0036339, 0.0036459125, 0.00366485, 0.0036882625, 0.0037156249999999997, 0.0037462374999999997, 0.0037875499999999998, 0.0038241875, 0.0038637, 0.0039045, 0.0039459874999999995, 0.0039884125, 0.004033124999999999, 0.0040762624999999995, 0.0041364625, 0.004200525, 0.0042620125, 0.004327325, 0.0044533875, 0.0045544374999999995, 0.0047220874999999995, 0.004831825, 0.0050000374999999994, 0.0051061125, 0.00520615, 0.0053232999999999996, 0.0054230625, 0.0055189875, 0.0056468874999999995, 0.0057696125, 0.0059131374999999995, 0.0060855125, 0.0062898375, 0.0065187249999999995, 0.00681645, 0.0071885, 0.0076144375, 0.0080546375, 0.0085025625, 0.0089830875, 0.0095602625, 0.01024395, 0.0110518375, 0.012105875, 0.0135318375, 0.015571375, 0.0188555875, 0.0250625375, 0.0417619125, 0.0370965625, 0.0255127375, 0.0178803, 0.014078175, 0.0118419875, 0.0103363, 0.009149125, 0.008374375, 0.0077541749999999994, 0.007196937499999999, 0.006757699999999999, 0.006424475, 0.006133624999999999, 0.005865537499999999, 0.0056292, 0.0054223875, 0.0052521875, 0.0051021625, 0.0049691875, 0.004847275, 0.0047343375, 0.004634075, 0.004542775, 0.004455375, 0.0043829125, 0.0043194875, 0.00426055, 0.004197025, 0.004150775, 0.0041064625, 0.004062725, 0.0040282875, 0.004001875, 0.0039816, 0.003968075, 0.0039587875, 0.00395545, 0.00396025, 0.0039688125, 0.0039852375, 0.0040066875, 0.004035775, 0.00406935, 0.0041077375, 0.0041456374999999995, 0.00418535, 0.004225225]] ("data 2"), error in (no error)="error in (no error)") -> (queue out=w60:refnum<queue>, error out=w63:errorcluster)  [unwired: 3 in, 1 out]
      n22 = while {
        tunnel: w53 -> [w124]
        tunnel: w52 -> [w123]
        shift-right: [w119] -> w62
        shift-left: w60 -> [w122]
        shift-right: [w118] -> w61
        shift-left: w63 -> [w120]
        tunnel: [w116] -> w57
        tunnel: [w115] -> w56
        tunnel: w48 -> [w114]
        tunnel: [w110] -> w51
        i -> [w112]
        stop <- w110 stop-if-true
        n23 = for {
          tunnel: w124 -> [w134] mode=indexing
          tunnel: w123 -> [w133] mode=indexing
          tunnel: [w131] -> w121 mode=indexing
          tunnel: [w128] -> w116 mode=indexing
          tunnel: [w126] -> w115 mode=indexing
          tunnel: w114 -> [w130] mode=indexing
          tunnel: [w125] -> _ mode=indexing
          n24 = call-poly <vilib>:"DAQmx Read.vi"("task/channels in"=w134, "number of samples per channel"=w130, "timeout"=1800.0, "error in"=w133) -> ("task out"=w129:refnum<k21>, "data"=w131:dbl[], "error out"=w127:errorcluster)  [unwired: 9 in]
          n25 = call <vilib>:"DAQmx Is Task Done.vi"("task/channels in"=w129, "error in"=w127) -> ("task out"=w128:refnum<k21>, "task done?"=w125:bool, "error out"=w126:errorcluster)  [unwired: 11 in]
        }
        n26 = Enqueue Element(queue=w122, element=w121, error in (no error)=w120) -> (queue out=w119:refnum<queue>, error out=w118:errorcluster)  [unwired: 1 in, 1 out]
        n27 = call "STOP FGV.vi"("Enum"=enum16{"Initialize", "Read", "Write"}."Read") -> ("OUT"=w111:bool)  [unwired: 9 in, 1 out]
        n28 = And(x=TRUE, y=w111) -> (x .and. y?=w110:bool)
        n29 = Wait (ms)(milliseconds to wait=u32 0) -> ()  [unwired: 1 out]
        "Counter Producer" <- w112
      }
      n30 = while {
        tunnel: w60 -> [w101]
        tunnel: "PPR Array" -> [w93]
        i -> [w88]
        stop <- w100 stop-if-true
        n31 = Dequeue Element(queue=w101) -> (element=w89:dbl[][], error out=w100:errorcluster)  [unwired: 2 in, 2 out]
        n32 = Transpose 2D Array(2D array=w89) -> (transposed array=→"data":dbl[][])
        n33 = for {
          tunnel: [w106] -> w91 mode=indexing
          tunnel: w93 -> [w103] mode=indexing
          tunnel: w89 -> [w104] mode=indexing
          n34 = Array Subset(array=w104, length=w103) -> (w102:dbl[])  [unwired: 1 in]
          "Array" <- w102
          n35 = call-poly <vilib>:"Mean.vi"("X"=w102) -> ("mean"=w108:dbl)  [unwired: 1 out]
          n36 = Multiply(x=w108, y=w103) -> (x*y=w105:dbl)
          n37 = Divide(x=60.0, y=w105) -> (x/y=w106:dbl)
          "PPR" <- w103
        }
        n38 = Index Array(array=w91, index #1=0 ("index")) -> (element #1=w92:dbl, element #2=→"Mean RPM_2SPD_OT":dbl)  [unwired: 1 in]
        "Mean RPM_DRVLN" <- w92
        n39 = Not A Number/Path/Refnum?(number/path/refnum=w92) -> (NaN/Path/Refnum?=w97:bool)
        n40 = Less?(x=w92, y=10.0) -> (x < y?=w96:bool)
        n41 = Or(x=w97, y=w96) -> (x .or. y?=w95:bool)
        n42 = property on="Mean RPM_DRVLN" class="DigNum (strict)"("Blinking"=w95) -> ()  [unwired: 2 in, 2 out]
        n43 = call "FGV arrDoubleNumeric.vi"("Array IN"=w91, "Enum"=enum16{"Read", "Write"}."Write") -> ()  [unwired: 8 in, 2 out]
        "Counter Consumer" <- w88
      }
      n44 = Release Queue(queue=w62, error in (no error)=w61) -> (error out=w58:errorcluster)  [unwired: 1 in, 2 out]
      "error out" <- w58
      n45 = case shown="True" w51 {
        tunnel: w57 -> [_ w66]
        tunnel: w56 -> [_ w65]
        frame False {
        }
        frame True {
          n46 = for {
            tunnel: w66 -> [w70] mode=indexing
            tunnel: w65 -> [w71] mode=indexing
            n47 = call <vilib>:"DAQmx Stop Task.vi"("task/channels in"=w70, "error in"=w71) -> ("task out"=w69:refnum<k21>, "error out"=w68:errorcluster)  [unwired: 12 in]
            n48 = call <vilib>:"DAQmx Clear Task.vi"("task in"=w69, "error in"=w68) -> ("error out"=w67:errorcluster)  [unwired: 13 in]
            n49 = call <vilib>:"Clear Errors.vi"("error in (no error)"=w67) -> ()  [unwired: 5 in, 2 out]
          }
        }
      }
      n50 = call <vilib>:"Simple Error Handler.vi"("error in (no error)"=w58) -> ()  [unwired: 4 in, 5 out]
    }
  }
  n51 = while {
    tunnel: w45 -> [w407]
    tunnel: w46 -> [w406]
    tunnel: [w405] -> w44
    tunnel: 200 ("number of samples per channel") -> [w216]
    tunnel: w30 -> [w259]
    tunnel: w29 -> [w258]
    tunnel: [w257] -> w24
    tunnel: [w256] -> w23
    shift-right: [w239] -> w19
    shift-left: w17 -> [w242]
    shift-right: [w238] -> w18
    shift-left: w20 -> [w241]
    tunnel: "Rate" -> [w224]
    tunnel: [w214] -> w5
    tunnel: [w213] -> w4
    tunnel: w2 -> [w212]
    i -> [w221]
    stop <- w402 stop-if-true
    w403 = 10.0  # timeout
    # "RPS"
    # "107 teeth"
    # "127 teeth"
    # "rpm"
    # "N·m"
    # "loop time (s)"
    # "=0 at multiples of 150 (30 seconds)"
    # "Note:  Hoffer 1-5 V = 0-60 gpm"
    # "Note: APD7580 F-V ±5 V = 0-5607.48 rpm"
    # "Note:  Omega TXDIN70  1-5V = 0-200 °C"
    # "Note: Kistler RAJ44A   0-5V = 0-10 bar a"
    # "Note: Kistler RAJ44A   0-5V = 0-10 bar a"
    # "Note:  Kistler RAJ44A   0-5V = 0-5 bar a"
    # "Note:  Omega TQ513   0-5V = ±1000in-lb"
    # "7."
    n52 = Divide(x=w216, y=w224) -> (x/y=w223:dbl)
    n53 = Divide(x=w216, y=100.0) -> (x/y=w244:dbl)
    n54 = call "FGV arrDoubleNumeric.vi"("Enum"=enum16{"Read", "Write"}."Read") -> ("Array OUT"=w274:dbl[])  [unwired: 9 in, 1 out]
    n55 = Index Array(array="LV_CMD_2SPD_OIL_SLND", index=0) -> (element=w253:bool)
    n56 = Divide(x="switch_time (s)", y=w223) -> (x/y=w220:dbl)
    "switch_counts" <- w220
    n57 = call-poly <vilib>:"DAQmx Read.vi"("task/channels in"=w407, "number of samples per channel"=w216, "timeout"=w403, "error in"=w406) -> ("task out"=w405:refnum<k21>, "data"=w211:waveform(dbl)[], "error out"=w215:errorcluster)  [unwired: 9 in]
    n58 = call-poly <vilib>:"DAQmx Read.vi"("task/channels in"=w212, "number of samples per channel"=w216, "error in"=w215) -> ("task out"=w213:refnum<k21>, "data"=w210:waveform(dbl)[], "error out"=w214:errorcluster)  [unwired: 10 in]
    n59 = call-poly <vilib>:"DAQmx Write.vi"("task/channels in"=w259, "data"="LV_CMD_2SPD_OIL_SLND", "timeout"=10.0, "error in"=w258) -> ("task out"=w257:refnum<k21>, "error out"=w256:errorcluster)  [unwired: 9 in, 1 out]
    n60 = Index Array(array=w274, index #1=0 ("index"), index #2=1 ("index")) -> (element #1=w273:dbl, element #2=w260:dbl)
    n61 = xnode "Formula"("X1"=w221, "X2"=w220) -> ("Result"=w219:dbl)  [unwired: 1 in, 1 out]
    n62 = Boolean To (0,1)(Boolean=w253) -> (0, 1=w245:i16)
    n63 = Build Array (concatenate)(w211, w210) -> (w209:waveform(dbl)[])
    n64 = Multiply(x=1.0, y=w273) -> (x*y=w309:dbl)
    n65 = Multiply(x=1.0, y=w260) -> (x*y=w268:dbl)
    n66 = Initialize Array("Data Tag", w244) -> (w277:dbl[])
    n67 = Initialize Array(w245, w244) -> (w237:i16[])
    n68 = Greater Than 0?(x=w221) -> (x > 0?=w226:bool)
    n69 = Equal To 0?(x=w219) -> (x = 0?=w225:bool)
    n70 = disable-structure shown="Disabled" {
      frame Disabled {
        n71 = expression code="mod(x,150)"() -> ()  [unwired: 1 in, 1 out]
      }
      frame Enabled {
      }
    }
    n72 = Initialize Array(w309, w244) -> (w321:dbl[])
    n73 = Initialize Array(w268, w244) -> (w267:dbl[])
    n74 = And(x=w226, y=w225) -> (x .and. y?=w227:bool)
    n75 = call-poly <vilib>:"Index Waveform Array.vi"("index"=0, "waveform array"=w209) -> ("waveform"=w310:waveform(dbl))  [unwired: 8 in, 1 out]
    n76 = case shown="True" w227 {
      tunnel: "LV_CMD_2SPD_OIL_SLND" -> [_ w419]
      frame False {
      }
      frame True {
        n77 = Not(x=w419) -> (.not. x?=w418:bool[])
        n78 = local write "LV_CMD_2SPD_OIL_SLND"(w418) -> ()
      }
    }
    n79 = for {
      tunnel: w209 -> [w422] mode=indexing
      tunnel: [w421] -> w141 mode=indexing
      tunnel: w310 -> [w420]
      # "Averaging"
      n80 = call "Sample Compression"("Signals"=w422) -> ("Mean"=w423:dynamicdata)  [unwired: 8 in, 2 out]
      n81 = call "Convert from Dynamic Data"("Dynamic Data Type"=w423) -> ("Array"=w425:dbl[])  [unwired: 3 in]
      n82 = Bundle By Name(cluster=w420, "Y"=w425, "dt"=0.1) -> (w421:waveform(dbl))
    }
    "data 2" <- w141
    n83 = call-poly <vilib>:"Index Waveform Array.vi"("index"=5, "waveform array"=w141) -> ("error out"=w306:errorcluster, "waveform"=w246:waveform(dbl))  [unwired: 8 in]
    n84 = call-poly <vilib>:"Index Waveform Array.vi"("index"=1, "waveform array"=w141) -> ("error out"=w375:errorcluster, "waveform"=w374:waveform(dbl))  [unwired: 8 in]
    n85 = call-poly <vilib>:"Index Waveform Array.vi"("index"=2, "waveform array"=w141) -> ("error out"=w366:errorcluster, "waveform"=w367:waveform(dbl))  [unwired: 8 in]
    n86 = call-poly <vilib>:"Index Waveform Array.vi"("index"=9, "waveform array"=w141) -> ("error out"=w165:errorcluster, "waveform"=w164:waveform(dbl))  [unwired: 8 in]
    n87 = call-poly <vilib>:"Index Waveform Array.vi"("index"=7, "waveform array"=w141) -> ("error out"=w198:errorcluster, "waveform"=w197:waveform(dbl))  [unwired: 8 in]
    n88 = call-poly <vilib>:"Index Waveform Array.vi"("index"=11, "waveform array"=w141) -> ("error out"=w146:errorcluster, "waveform"=w145:waveform(dbl))  [unwired: 8 in]
    n89 = call-poly <vilib>:"Index Waveform Array.vi"("index"=8, "waveform array"=w141) -> ("error out"=w189:errorcluster, "waveform"=w190:waveform(dbl))  [unwired: 8 in]
    n90 = call-poly <vilib>:"Index Waveform Array.vi"("index"=6, "waveform array"=w141) -> ("error out"=w396:errorcluster, "waveform"=w397:waveform(dbl))  [unwired: 8 in]
    n91 = call-poly <vilib>:"Index Waveform Array.vi"("index"=0, "waveform array"=w141) -> ("error out"=w230:errorcluster, "waveform"=w231:waveform(dbl))  [unwired: 8 in]
    n92 = call-poly <vilib>:"Index Waveform Array.vi"("index"=3, "waveform array"=w141) -> ("error out"=w350:errorcluster, "waveform"=w349:waveform(dbl))  [unwired: 8 in]
    n93 = call-poly <vilib>:"Index Waveform Array.vi"("index"=4, "waveform array"=w141) -> ("error out"=w341:errorcluster, "waveform"=w342:waveform(dbl))  [unwired: 8 in]
    n94 = Bundle By Name(cluster=w231, "Y"=w321) -> (w292:waveform(dbl))
    n95 = Bundle By Name(cluster=w246, "Y"=w277) -> (w283:waveform(dbl))
    n96 = Bundle By Name(cluster=w231, "Y"=w267) -> (w269:waveform(dbl))
    n97 = Bundle By Name(cluster=w246, "Y"=w237) -> (w247:waveform(dbl))
    n98 = Set Waveform Attribute(4:w306, 5:"VFr_OIL_2SPD_IN" ("name"), 6:"NI_ChannelName" ("name"), 7:w246) -> (3:w304:waveform(dbl))  [unwired: 2 out]
    n99 = Set Waveform Attribute(4:w375, 5:"P_2SPD_VENT" ("name"), 6:"NI_ChannelName" ("name"), 7:w374) -> (3:w378:waveform(dbl))  [unwired: 2 out]
    n100 = Set Waveform Attribute(4:w366, 5:"P_OIL_2SPD_IN" ("name"), 6:"NI_ChannelName" ("name"), 7:w367) -> (3:w363:waveform(dbl))  [unwired: 2 out]
    n101 = Set Waveform Attribute(4:w165, 5:"T_2SPD_OIL_OT" ("name"), 6:"NI_ChannelName" ("name"), 7:w164) -> (3:w168:waveform(dbl))  [unwired: 2 out]
    n102 = Set Waveform Attribute(4:w198, 5:"TRQ_2SPD_OT" ("name"), 6:"NI_ChannelName" ("name"), 7:w197) -> (3:w201:waveform(dbl))  [unwired: 2 out]
    n103 = Set Waveform Attribute(4:w146, 5:"TRQ_T22_2SPD_INPUT_PULLEY" ("name"), 6:"NI_ChannelName" ("name"), 7:w145) -> (3:w149:waveform(dbl))  [unwired: 2 out]
    n104 = Set Waveform Attribute(4:w189, 5:"RPM_2SPD_IN_FV" ("name"), 6:"NI_ChannelName" ("name"), 7:w190) -> (3:w186:waveform(dbl))  [unwired: 2 out]
    n105 = Set Waveform Attribute(4:w396, 5:"TRQ_2SPD_DRVLN_OT" ("name"), 6:"NI_ChannelName" ("name"), 7:w397) -> (3:w393:waveform(dbl))  [unwired: 2 out]
    n106 = Set Waveform Attribute(4:w350, 5:"P_OIL_2SPD_SLND_OT" ("name"), 6:"NI_ChannelName" ("name"), 7:w349) -> (3:w353:waveform(dbl))  [unwired: 2 out]
    n107 = Set Waveform Attribute(4:w341, 5:"T_2SPD_OIL_IN" ("name"), 6:"NI_ChannelName" ("name"), 7:w342) -> (3:w338:waveform(dbl))  [unwired: 2 out]
    n108 = Set Waveform Attribute(4:w230, 5:"RPM_2SPD_OT_FV" ("name"), 6:"NI_ChannelName" ("name"), 7:w231) -> (3:w234:waveform(dbl))  [unwired: 2 out]
    n109 = Set Waveform Attribute(5:"RPM_DRVLN_6602" ("name"), 6:"NI_ChannelName" ("name"), 7:w292) -> (3:w326:waveform(dbl))  [unwired: 1 in, 2 out]
    n110 = Set Waveform Attribute(5:"RPM_2SPD_OT_6602" ("name"), 6:"NI_ChannelName" ("name"), 7:w269) -> (3:w263:waveform(dbl))  [unwired: 1 in, 2 out]
    n111 = Set Waveform Attribute(5:"DataTag" ("name"), 6:"NI_ChannelName" ("name"), 7:w283) -> (3:w281:waveform(dbl))  [unwired: 1 in, 2 out]
    n112 = Set Waveform Attribute(5:"LV_CMD_2SPD_OIL_SLND" ("name"), 6:"NI_ChannelName" ("name"), 7:w247) -> (3:w249:waveform(dbl))  [unwired: 1 in, 2 out]
    n113 = Set Waveform Attribute(5:"gpm" ("name"), 6:"NI_UnitDescription" ("name"), 7:w304) -> (3:w302:waveform(dbl))  [unwired: 1 in, 2 out]
    n114 = Set Waveform Attribute(5:"bar_a" ("name"), 6:"NI_UnitDescription" ("name"), 7:w378) -> (3:w381:waveform(dbl))  [unwired: 1 in, 2 out]
    n115 = Set Waveform Attribute(5:"bar_a" ("name"), 6:"NI_UnitDescription" ("name"), 7:w363) -> (3:w360:waveform(dbl))  [unwired: 1 in, 2 out]
    n116 = Set Waveform Attribute(5:"deg_C" ("name"), 6:"NI_UnitDescription" ("name"), 7:w168) -> (3:w171:waveform(dbl))  [unwired: 1 in, 2 out]
    n117 = Set Waveform Attribute(5:"N·m" ("name"), 6:"NI_UnitDescription" ("name"), 7:w201) -> (3:w204:waveform(dbl))  [unwired: 1 in, 2 out]
    n118 = Set Waveform Attribute(5:"N·m" ("name"), 6:"NI_UnitDescription" ("name"), 7:w149) -> (3:w152:waveform(dbl))  [unwired: 1 in, 2 out]
    n119 = Set Waveform Attribute(5:"rpm" ("name"), 6:"NI_UnitDescription" ("name"), 7:w186) -> (3:w183:waveform(dbl))  [unwired: 1 in, 2 out]
    n120 = Set Waveform Attribute(5:"N·m" ("name"), 6:"NI_UnitDescription" ("name"), 7:w393) -> (3:w390:waveform(dbl))  [unwired: 1 in, 2 out]
    n121 = Set Waveform Attribute(5:"bar_a" ("name"), 6:"NI_UnitDescription" ("name"), 7:w353) -> (3:w356:waveform(dbl))  [unwired: 1 in, 2 out]
    n122 = Set Waveform Attribute(5:"deg_C" ("name"), 6:"NI_UnitDescription" ("name"), 7:w338) -> (3:w335:waveform(dbl))  [unwired: 1 in, 2 out]
    n123 = Set Waveform Attribute(5:"rpm" ("name"), 6:"NI_UnitDescription" ("name"), 7:w234) -> (3:w229:waveform(dbl))  [unwired: 1 in, 2 out]
    n124 = Set Waveform Attribute(5:"rpm" ("name"), 6:"NI_UnitDescription" ("name"), 7:w326) -> (3:w155:waveform(dbl))  [unwired: 1 in, 2 out]
    n125 = Set Waveform Attribute(5:"rpm" ("name"), 6:"NI_UnitDescription" ("name"), 7:w263) -> (3:w154:waveform(dbl))  [unwired: 1 in, 2 out]
    n126 = Set Waveform Attribute(5:"none" ("name"), 6:"NI_UnitDescription" ("name"), 7:w281) -> (3:w275:waveform(dbl))  [unwired: 1 in, 2 out]
    n127 = Set Waveform Attribute(5:"boolean" ("name"), 6:"NI_UnitDescription" ("name"), 7:w249) -> (3:w243:waveform(dbl))  [unwired: 1 in, 2 out]
    n128 = Unbundle By Name(w155) -> ("Y"=w323:dbl[])
    n129 = Unbundle By Name(w154) -> ("Y"=w266:dbl[])
    n130 = Multiply(x="RPM_IN rpm/V", y="DRVLN_PULLEY_RATIO") -> (x*y=→"CALC_RPM_2SPD_IN_FV":dbl)
    n131 = call-poly <vilib>:"Mean.vi"("X"=w323) -> ("mean"=w217:dbl)  [unwired: 1 out]
    "RPM_DRVLN_6602" <- w217
    n132 = call <vilib>:"Waveform Scale and Offset.vi"("scale"="F2 gpm/V", "offset"="offset_F2", "waveform in"=w302) -> ("waveform out"=w298:waveform(dbl))  [unwired: 7 in, 1 out]
    n133 = call-poly <vilib>:"Mean.vi"("X"=w266) -> ("mean"=→"RPM_2SPD_OT_6602":dbl)  [unwired: 1 out]
    n134 = call <vilib>:"Waveform Scale and Offset.vi"("scale"="P1 bar_a/V", "offset"="offset_P1", "waveform in"=w381) -> ("waveform out"=w320:waveform(dbl))  [unwired: 7 in, 1 out]
    n135 = call <vilib>:"Waveform Scale and Offset.vi"("scale"="P2 bar_a/V", "offset"="offset_P2", "waveform in"=w360) -> ("waveform out"=w319:waveform(dbl))  [unwired: 7 in, 1 out]
    n136 = call <vilib>:"Waveform Scale and Offset.vi"("scale"="T2 °C/V", "offset"="offset_T2", "waveform in"=w171) -> ("waveform out"=w160:waveform(dbl))  [unwired: 7 in, 1 out]
    n137 = call <vilib>:"Waveform Scale and Offset.vi"("scale"="N·m/V", "offset"="offset TRQ_OT", "waveform in"=w204) -> ("waveform out"=w180:waveform(dbl))  [unwired: 7 in, 1 out]
    n138 = call <vilib>:"Waveform Scale and Offset.vi"("scale"="(N·m)/V TRQ_IN", "offset"="offset_TRQ_IN", "waveform in"=w152) -> ("waveform out"=w138:waveform(dbl))  [unwired: 7 in, 1 out]
    n139 = call <vilib>:"Waveform Scale and Offset.vi"("scale"="RPM_IN rpm/V", "offset"="offset RPM_IN", "waveform in"=w183) -> ("waveform out"=w181:waveform(dbl))  [unwired: 7 in, 1 out]
    n140 = call <vilib>:"Waveform Scale and Offset.vi"("scale"="RPM_OT/V", "offset"="offset_RPM1", "waveform in"=w229) -> ("waveform out"=w139:waveform(dbl))  [unwired: 7 in, 1 out]
    n141 = call <vilib>:"Waveform Scale and Offset.vi"("scale"="P3 bar_g/V", "offset"="offset_P3", "waveform in"=w356) -> ("waveform out"=w318:waveform(dbl))  [unwired: 7 in, 1 out]
    n142 = call <vilib>:"Waveform Scale and Offset.vi"("scale"="T1 °C/V", "offset"="offset_T1", "waveform in"=w335) -> ("waveform out"=w317:waveform(dbl))  [unwired: 7 in, 1 out]
    n143 = call <vilib>:"Waveform Scale and Offset.vi"("scale"="(N·m)/V DRVLN", "offset"="offset_TRQ_DRVLN", "waveform in"=w390) -> ("waveform out"=w153:waveform(dbl))  [unwired: 7 in, 1 out]
    n144 = Not A Number/Path/Refnum?(number/path/refnum=w217) -> (NaN/Path/Refnum?=w315:bool)
    n145 = Less?(x=w217, y=0.0) -> (x < y?=w316:bool)
    n146 = Unbundle By Name(w138) -> ("Y"=w140:dbl[])
    n147 = Unbundle By Name(w298) -> ("Y"=w297:dbl[])
    n148 = Unbundle By Name(w320) -> ("Y"=w382:dbl[])
    n149 = Unbundle By Name(w319) -> ("Y"=w359:dbl[])
    n150 = Unbundle By Name(w160) -> ("Y"=w173:dbl[])
    n151 = Unbundle By Name(w180) -> ("Y"=w205:dbl[])
    n152 = Or(x=w315, y=w316) -> (x .or. y?=w313:bool)
    n153 = Unbundle By Name(w181) -> ("Y"=w182:dbl[])
    n154 = Unbundle By Name(w139) -> ("Y"=w332:dbl[])
    n155 = Unbundle By Name(w318) -> ("Y"=w358:dbl[])
    n156 = Unbundle By Name(w317) -> ("Y"=w333:dbl[])
    n157 = call-poly <vilib>:"Mean.vi"("X"=w140) -> ("mean"=w135:dbl)  [unwired: 1 out]
    "TRQ_T22_2SPD_INPUT_PULLEY" <- w135
    n158 = call-poly <vilib>:"Mean.vi"("X"=w297) -> ("mean"=→"F2":dbl)  [unwired: 1 out]
    n159 = call-poly <vilib>:"Mean.vi"("X"=w382) -> ("mean"=w295:dbl)  [unwired: 1 out]
    "P1" <- w295
    n160 = call-poly <vilib>:"Mean.vi"("X"=w359) -> ("mean"=w296:dbl)  [unwired: 1 out]
    "P2" <- w296
    n161 = call-poly <vilib>:"Mean.vi"("X"=w173) -> ("mean"=→"T2":dbl)  [unwired: 1 out]
    n162 = call-poly <vilib>:"Mean.vi"("X"=w205) -> ("mean"=w193:dbl)  [unwired: 1 out]
    "TRQ_2SPD_OT (N·m)" <- w193
    n163 = property on="RPM_DRVLN_6602" class="DigNum (strict)"("Blinking"=w313) -> ()  [unwired: 2 in, 2 out]
    n164 = call-poly <vilib>:"Mean.vi"("X"=w182) -> ("mean"=w136:dbl)  [unwired: 1 out]
    "RPM_2SPD_IN_FV" <- w136
    n165 = call-poly <vilib>:"Mean.vi"("X"=w332) -> ("mean"=w137:dbl)  [unwired: 1 out]
    "RPM_2SPD_OT_FV" <- w137
    n166 = call-poly <vilib>:"Mean.vi"("X"=w358) -> ("mean"=→"P3":dbl)  [unwired: 1 out]
    n167 = call-poly <vilib>:"Mean.vi"("X"=w333) -> ("mean"=→"T1":dbl)  [unwired: 1 out]
    n168 = Divide(x=w137, y=60.0) -> (x/y=w176:dbl)
    n169 = Subtract(x=w296, y=w295) -> (x-y=→"delta-P":dbl)
    n170 = Multiply(x=6.283185307179586, y=w176) -> (x*y=w207:dbl)
    n171 = Divide(x=w273, y=60.0) -> ()  [unwired: 1 out]
    n172 = Multiply(x=w193, y=w207) -> (x*y=→"Power_OT (W)":dbl)
    n173 = Unbundle By Name(w153) -> ("Y"=w398:dbl[])
    n174 = Unbundle By Name(w214) -> ("status"=w404:bool)
    n175 = Divide(x=w136, y=60.0) -> (x/y=w174:dbl)
    n176 = call-poly <vilib>:"Mean.vi"("X"=w398) -> ("mean"=→"TRQ_2SPD_DRVLN_OT (N·m)":dbl)  [unwired: 1 out]
    n177 = Divide(x=w137, y=w136) -> (x/y=w178:dbl)
    "rpm_out/rpm_in" <- w178
    n178 = Initialize Array(w178, w244) -> (w291:dbl[])
    n179 = Bundle By Name(cluster=w246, "Y"=w291) -> (w285:waveform(dbl))
    n180 = Set Waveform Attribute(5:"RPM_RATIO" ("name"), 6:"NI_ChannelName" ("name"), 7:w285) -> (3:w287:waveform(dbl))  [unwired: 1 in, 2 out]
    n181 = Set Waveform Attribute(5:"ratio" ("name"), 6:"NI_UnitDescription" ("name"), 7:w287) -> (3:w284:waveform(dbl))  [unwired: 1 in, 2 out]
    n182 = Build Array(w180, w181, w153, w320, w319, w318, w317, w160, w138, w139, w155, w154, w298, w284, w275, w243) -> (w240:waveform(dbl)[])
    "Waveform Chart" <- w240
    n183 = Multiply(x=6.283185307179586, y=w174) -> (x*y=w384:dbl)
    n184 = Enqueue Element(queue=w242, element=w240, error in (no error)=w241) -> (queue out=w239:refnum<queue>, error out=w238:errorcluster)  [unwired: 1 in, 1 out]
    n185 = Or(x=w404, y="stop") -> (x .or. y?=w402:bool)
    n186 = Multiply(x=w135, y=w384) -> (x*y=→"Power_IN (W)":dbl)
    n187 = call "STOP FGV.vi"("IN"="stop", "Enum"=enum16{"Initialize", "Read", "Write"}."Write") -> ()  [unwired: 8 in, 2 out]
    n188 = Wait (ms)(milliseconds to wait=u32 5) -> ()  [unwired: 1 out]
    "AI Producer Iterations" <- w221
  }
  n189 = while {
    tunnel: w17 -> [w435]
    i -> [w434]
    stop <- w426 stop-if-true
    n190 = Dequeue Element(queue=w435) -> (element=w429:waveform(dbl)[], error out=w427:errorcluster)  [unwired: 2 in, 2 out]
    n191 = call "Select_Waveform_By_Name_rev_160122_A.vi"("Array"=string[] ["DataTag"], "Waveform Array"=w429) -> ("Array 2"=w432:waveform(dbl)[])  [unwired: 9 in]
    n192 = call-poly <vilib>:"Index Waveform Array.vi"("waveform array"=w432) -> ("waveform"=w431:waveform(dbl))  [unwired: 9 in, 1 out]
    n193 = Unbundle By Name(w431) -> ("Y"=w430:dbl[])
    n194 = Index Array(array=w430) -> (element=w428:dbl)  [unwired: 1 in]
    n195 = call "Record Continuous Tags Rev 170821_A.vi"("Run Letter"="Run Letter", "path"="path", "Waveform Array In"=w429, "Force Record"="Force Record", "Main Count"=w434, "Num_Blocks"="Num_Blocks", "Data Tag"=w428) -> ("Record Cmd"=w441:bool, "Recorded Blocks"=→"Recorded Blocks":dbl)  [unwired: 2 in, 1 out]
    "Recording" <- w441
    n196 = call <vilib>:"Boolean Crossing PtByPt.vi"("direction"=enum16{"either", "false-true", "true-false"}."true-false", "input"=w441) -> ("crossing"=w442:bool)  [unwired: 1 in]
    n197 = case shown="True" w442 {
      frame False {
      }
      frame True {
        n198 = local write "Data Tag"(99.0 ("y")) -> ()
      }
    }
    n199 = Unbundle By Name(w427) -> ("status"=w426:bool)
    "AI Consumer Iterations" <- w434
  }
  n200 = Release Queue(queue=w19, error in (no error)=w18) -> ()  [unwired: 1 in, 3 out]
  n201 = call <vilib>:"DAQmx Clear Task.vi"("task in"=w4, "error in"=w5) -> ("error out"=w3:errorcluster)  [unwired: 13 in]
  n202 = call <vilib>:"DAQmx Stop Task.vi"("task/channels in"=w24, "error in"=w23) -> ("task out"=w26:refnum<k21>, "error out"=w25:errorcluster)  [unwired: 12 in]
  n203 = call <vilib>:"DAQmx Clear Task.vi"("task in"=w26, "error in"=w25) -> ("error out"=w28:errorcluster)  [unwired: 13 in]
  n204 = call <vilib>:"DAQmx Clear Task.vi"("task in"=w44, "error in"=w3) -> ("error out"=w47:errorcluster)  [unwired: 13 in]
  n205 = call <vilib>:"Simple Error Handler.vi"("type of dialog (OK msg:1)"=w27, "error in (no error)"=w28) -> ()  [unwired: 3 in, 5 out]
  n206 = call <vilib>:"Simple Error Handler.vi"("type of dialog (OK msg:1)"=w42, "error in (no error)"=w47) -> ()  [unwired: 3 in, 5 out]
